vi "Pose3d_RotationVectorToMatrix.vi"(11 "RotationVector":dbl[](array[numeric])) -> (3 "Rotation Matrix":T1)   [LabVIEW 2019, in "Trajectory_Library.lvlib"]
doc: "Transforms the pose by the given transformation and returns the new transformed pose. \"plus\" is the same as \"transformBy\"\n\nThe matrix multiplication is as follows\n [x_new] [cos, -sin, 0][transform.x]\n [y_new] += [sin, cos, 0][transform.y]\n [t_new] [0, 0, 1][transform.t]\n\nParameters:\n - IN POSE - The input POSE data structure\n - OTHER TRANSFORM - The transform to transform the pose by.\n\nReturn:\n - OUT POSE - The transformed pose."
uses:
  Pose3d_getTranslation3d.vi
  Pose3d_getRotation3d.vi
  Transform3d_GetTranslation3d.vi
  Transform3d_GetRotation3d.vi
  Translation3d_Plus.vi
  Translation3d_RotateBy.vi
  Pose3d_New_Trans3dRot3d.vi
  Rotation3d_Plus.vi
  Translation3d_Create.vi
  Rotation3d_GetQuaterion.vi
  Quaternion_New.vi
  Quaternion_Times.vi
  Quaternion_Inverse.vi
  Quaternion_Get_All.vi
  Rotation3d_RotateBy.vi
  Quaternion_Get_LVQuat.vi
  Quaternion_New_LVQuat.vi
  Quaternion_Equals.vi
  Rotation3d_Create_Quaternion.vi
  Quaternion_Normalize.vi
  Quaternion_New_Default.vi
  <vilib>/robotics/Kinematics/Multiply Quaternions.vi
  <vilib>/robotics/Kinematics/Multiply Quaternion by Quaternion.vi
  Trajectory_Library.lvlib
  <vilib>/Analysis/Matrix/Datatypes/RealMatrix.ctl
  <vilib>/Analysis/Matrix/NI_Matrix.lvlib
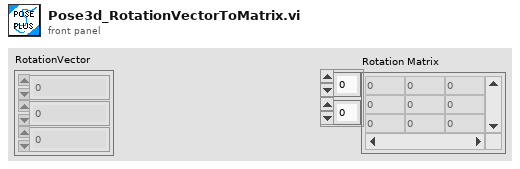
[diagram p1: front panel]
types:
  T1 = typedef "NI_Matrix.lvlib/RealMatrix.ctl" = dbl[][]
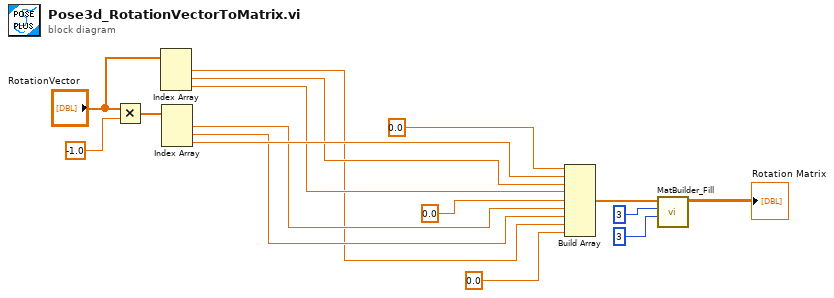
[diagram p0: block diagram]
diagram:
  n1 = Multiply(x="RotationVector", y=-1.0) -> (x*y=w8:dbl[])
  n2 = Index Array(array="RotationVector") -> (element #1=w1:dbl, element #2=w5:dbl, element #3=w4:dbl)  [unwired: 3 in]
  n3 = Index Array(array=w8) -> (element #1=w3:dbl, element #2=w2:dbl, element #3=w6:dbl)  [unwired: 3 in]
  n4 = Build Array(0.0 ("element"), w6, w5, w4, 0.0 ("element"), w3, w2, w1, 0.0 ("element")) -> (w13:dbl[])
  n5 = call "MatBuilder_Fill.vi"("Columns"=3, "Rows"=3, "Value List"=w13) -> ("output matrix"=→"Rotation Matrix":T1)  [unwired: 8 in]
